vi "notch_bandpass_ADS_filter.vi"(7 "Apply":bool, 8 "Filters":T1, 10 "Sampling frequency":dbl, 11 "Data in":dbl) -> (3 "Filtered x":dbl format="%0.2f")   [LabVIEW 2023]
uses:
  <vilib>/Analysis/3filter.llb/Filter Passband Type.ctl
  <vilib>/ptbypt/NI_PtbyPt.lvlib
  <vilib>/Analysis/NI_AALBase.lvlib
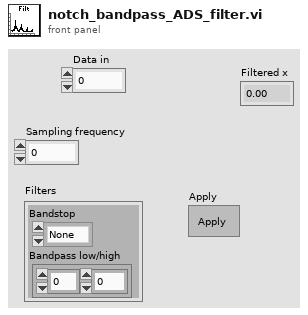
[diagram p1: front panel]
types:
  T1 = cluster{"Bandstop":enum16{"None", "50", "50 x N"}, "Bandpass low/high":cluster{i32, i32}}
  T2 = typedef "NI_AALBase.lvlib/Filter Passband Type.ctl" = enum32{"Lowpass", "Highpass", "Bandpass", "Bandstop"}
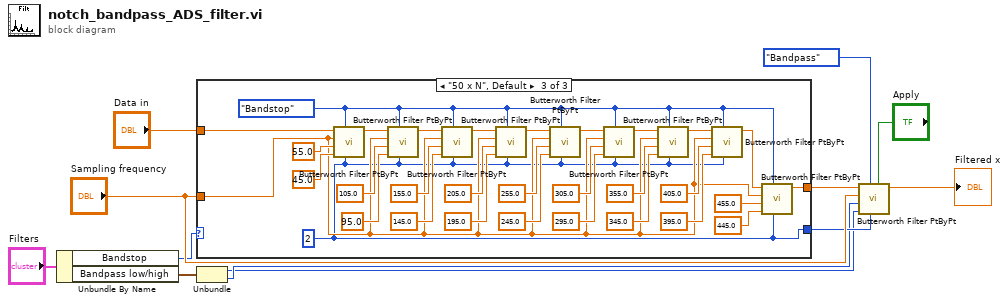
[diagram p0: block diagram]
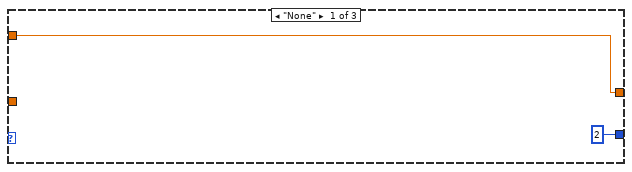
[diagram p2: hidden frame]
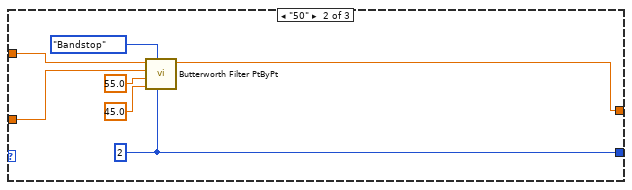
[diagram p3: hidden frame]
diagram:
  n1 = Unbundle By Name("Filters") -> ("Bandstop"=w5:enum16{"None", "50", "50 x N"}, "Bandpass low/high"=w4:cluster{i32, i32})
  n2 = case shown="\"50 x N\", Default" w5 {
    tunnel: "Sampling frequency" -> [_ w17 w26]
    tunnel: "Data in" -> [w14 w18 w25]
    tunnel: [w14 w16 w23] -> w11
    tunnel: [2 w15 w22] -> w9
    frame "None" {
    }
    frame "50" {
      w15 = 2
      n3 = call <vilib>:"Butterworth Filter PtByPt.vi"("order"=w15, "filter type"=Filter_Passband_Type."Bandstop", "low cutoff freq: fl"=45.0, "high cutoff freq: fh"=55.0, "sampling freq: fs"=w17, "x"=w18) -> ("Filtered x"=w16:dbl)  [unwired: 3 in, 1 out]
    }
    frame "50 x N", Default {
      w22 = 2
      w24 = Filter_Passband_Type."Bandstop" ("filter type")
      n4 = call <vilib>:"Butterworth Filter PtByPt.vi"("order"=w22, "filter type"=w24, "low cutoff freq: fl"=45.0, "high cutoff freq: fh"=55.0, "sampling freq: fs"=w26, "x"=w25) -> ("Filtered x"=w27:dbl)  [unwired: 3 in, 1 out]
      n5 = call <vilib>:"Butterworth Filter PtByPt.vi"("order"=w22, "filter type"=w24, "low cutoff freq: fl"=95.0, "high cutoff freq: fh"=105.0, "sampling freq: fs"=w26, "x"=w27) -> ("Filtered x"=w37:dbl)  [unwired: 3 in, 1 out]
      n6 = call <vilib>:"Butterworth Filter PtByPt.vi"("order"=w22, "filter type"=w24, "low cutoff freq: fl"=145.0, "high cutoff freq: fh"=155.0, "sampling freq: fs"=w26, "x"=w37) -> ("Filtered x"=w34:dbl)  [unwired: 3 in, 1 out]
      n7 = call <vilib>:"Butterworth Filter PtByPt.vi"("order"=w22, "filter type"=w24, "low cutoff freq: fl"=195.0, "high cutoff freq: fh"=205.0, "sampling freq: fs"=w26, "x"=w34) -> ("Filtered x"=w33:dbl)  [unwired: 3 in, 1 out]
      n8 = call <vilib>:"Butterworth Filter PtByPt.vi"("order"=w22, "filter type"=w24, "low cutoff freq: fl"=245.0, "high cutoff freq: fh"=255.0, "sampling freq: fs"=w26, "x"=w33) -> ("Filtered x"=w43:dbl)  [unwired: 3 in, 1 out]
      n9 = call <vilib>:"Butterworth Filter PtByPt.vi"("order"=w22, "filter type"=w24, "low cutoff freq: fl"=295.0, "high cutoff freq: fh"=305.0, "sampling freq: fs"=w26, "x"=w43) -> ("Filtered x"=w30:dbl)  [unwired: 3 in, 1 out]
      n10 = call <vilib>:"Butterworth Filter PtByPt.vi"("order"=w22, "filter type"=w24, "low cutoff freq: fl"=345.0, "high cutoff freq: fh"=355.0, "sampling freq: fs"=w26, "x"=w30) -> ("Filtered x"=w29:dbl)  [unwired: 3 in, 1 out]
      n11 = call <vilib>:"Butterworth Filter PtByPt.vi"("order"=w22, "filter type"=w24, "low cutoff freq: fl"=395.0, "high cutoff freq: fh"=405.0, "sampling freq: fs"=w26, "x"=w29) -> ("Filtered x"=w40:dbl)  [unwired: 3 in, 1 out]
      n12 = call <vilib>:"Butterworth Filter PtByPt.vi"("order"=w22, "filter type"=w24, "low cutoff freq: fl"=445.0, "high cutoff freq: fh"=455.0, "sampling freq: fs"=w26, "x"=w40) -> ("Filtered x"=w23:dbl)  [unwired: 3 in, 1 out]
    }
  }
  n13 = Unbundle(w4) -> (w7:i32, w8:i32)
  n14 = call <vilib>:"Butterworth Filter PtByPt.vi"("initialize"="Apply", "order"=w9, "filter type"=Filter_Passband_Type."Bandpass", "low cutoff freq: fl"=w7, "high cutoff freq: fh"=w8, "sampling freq: fs"="Sampling frequency", "x"=w11) -> ("Filtered x"=→"Filtered x":dbl)  [unwired: 2 in, 1 out]
